vi "Main.vi"(10 "VISA resource name":refnum<visa-resource-name>, 11 "Module Admin":refnum<class "Delacor_lib_QMH_Module Admin.lvclass">) -> ()   [LabVIEW 2018, in "SPIM7_CAM.lvlib"]
doc: "This template is based off of the Queued Message Handler design pattern and the Queued Message Handler project template that ships with LabVIEW.\n\nThe main difference is that the queue is private to this module and communication between modules is performed via Broadcast and Request events.\n\nRequest events are wrapped in public API methods and are handled in the Event Handling Loop (EHL) of this VI. Any module can register for Broadcast events sent by this module. The EHL generates messages based on user interface actions.\n\nThe Message Handling Loop (MHL) processes messages generated by the EHL, or by other messages. The messages are string values, so new messages can be added easily to the Message Cases case structure in the MHL. Each message cluster can also provide an optional value for Message Data, which is a variant that can be converted to whatever message-specific data is required.\n_____\nBased on DQMH Project Template 6.0.0.91."
uses:
  SPIM7_CAM.lvlib
  <vilib>/Delacor/Delacor QMH/Libraries/Module Admin_class/Delacor_lib_QMH_Module Admin.lvclass
  Module Data--cluster.ctl
  <vilib>/Delacor/Delacor QMH/Libraries/Message Queue_class/Delacor_lib_QMH_Message Queue.lvclass/Delacor_lib_QMH_Message Queue.ctl
  Stop Argument--cluster.ctl
  <vilib>/Delacor/Delacor QMH/Libraries/Module Admin_class/Delacor_lib_QMH_Module Admin.lvclass/Delacor_lib_QMH_Module Admin.ctl
  Open COM Argument--cluster.ctl
  Close COM Argument--cluster.ctl
  Read Pan angle Argument--cluster.ctl
  Read Pan angle (Reply Payload)--cluster.ctl
  Read TILT angle Argument--cluster.ctl
  Read TILT angle (Reply Payload)--cluster.ctl
  <vilib>/Utility/miscctls.llb/LVPointTypeDef.ctl
  <vilib>/Delacor/Delacor QMH/Libraries/Message Queue_class/Delacor_lib_QMH_Enqueue Message (Single).vi
  <vilib>/Delacor/Delacor QMH/Libraries/Module Admin_class/Delacor_lib_QMH_Get External Launch.vi
  <vilib>/Utility/error.llb/Error Cluster From Error Code.vi
  <vilib>/Instr/_visa.llb/VISA Configure Serial Port (Instr).vi
  <vilib>/ErrorRing/Error Ring.xnode
  <vilib>/Delacor/Delacor QMH/Libraries/Message Queue_class/Delacor_lib_QMH_Message Queue.lvclass
panel:
  out "error out":errorcluster
  out "Status":string
  in  "Simulate MHL Error":bool
  in  "Simulate EHL Error":bool
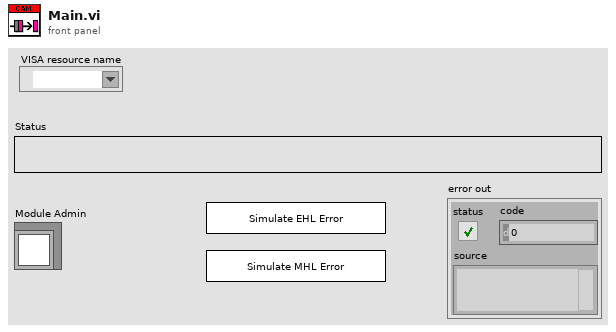
[diagram p1: front panel]
types:
  T1 = typedef "SPIM7_CAM.lvlib/Request Events--cluster.ctl" = cluster{"Stop Module":refnum<user-event>, "Show Panel":refnum<user-event>, "Hide Panel":refnum<user-event>, "Get Module Execution Status":refnum<user-event>, "Show Diagram":refnum<user-event>, "Open COM":refnum<user-event>, "Close COM":refnum<user-event>, "Read Pan angle":refnum<user-event>, "Read TILT angle":refnum<user-event>}
  T2 = typedef "SPIM7_CAM.lvlib/Module Data--cluster.ctl" = cluster{"Status":string, "VISA resource name":refnum<visa-resource-name>}
  T3 = enum32{"invalid lock state", "Not Locked", "Locked (No Password)", "Password-protected"}
  T4 = typedef "SPIM7_CAM.lvlib/Stop Argument--cluster.ctl" = cluster{"Origin":string, "Exit via Stop Module Req?":bool, "Wait for Module to stop?":bool}
  T5 = typedef "SPIM7_CAM.lvlib/Open COM Argument--cluster.ctl" = cluster{"baudrate":u32}
  T6 = typedef "SPIM7_CAM.lvlib/Close COM Argument--cluster.ctl" = cluster{"Boolean":bool}
  T7 = typedef "SPIM7_CAM.lvlib/Read Pan angle Argument--cluster.ctl" = cluster{"Wait Notifier":refnum<notifier>, "wait for reply":bool}
  T8 = typedef "SPIM7_CAM.lvlib/Read TILT angle Argument--cluster.ctl" = cluster{"Wait Notifier":refnum<notifier>, "wait for reply":bool}
  T9 = typedef "LVPointTypeDef.ctl" = cluster{"Horizontal":i16, "Vertical":i16}
  T10 = enum32{"Invalid", "Standard", "Closed", "Hidden", "Minimized", "Maximized"}
  T11 = typedef "SPIM7_CAM.lvlib/Read Pan angle (Reply Payload)--cluster.ctl" = cluster{"Pan angle":dbl, "Read Pan angle_error":errorcluster}
  T12 = typedef "SPIM7_CAM.lvlib/Read TILT angle (Reply Payload)--cluster.ctl" = cluster{"Tilt angle":dbl, "Read TILT angle_error":errorcluster}
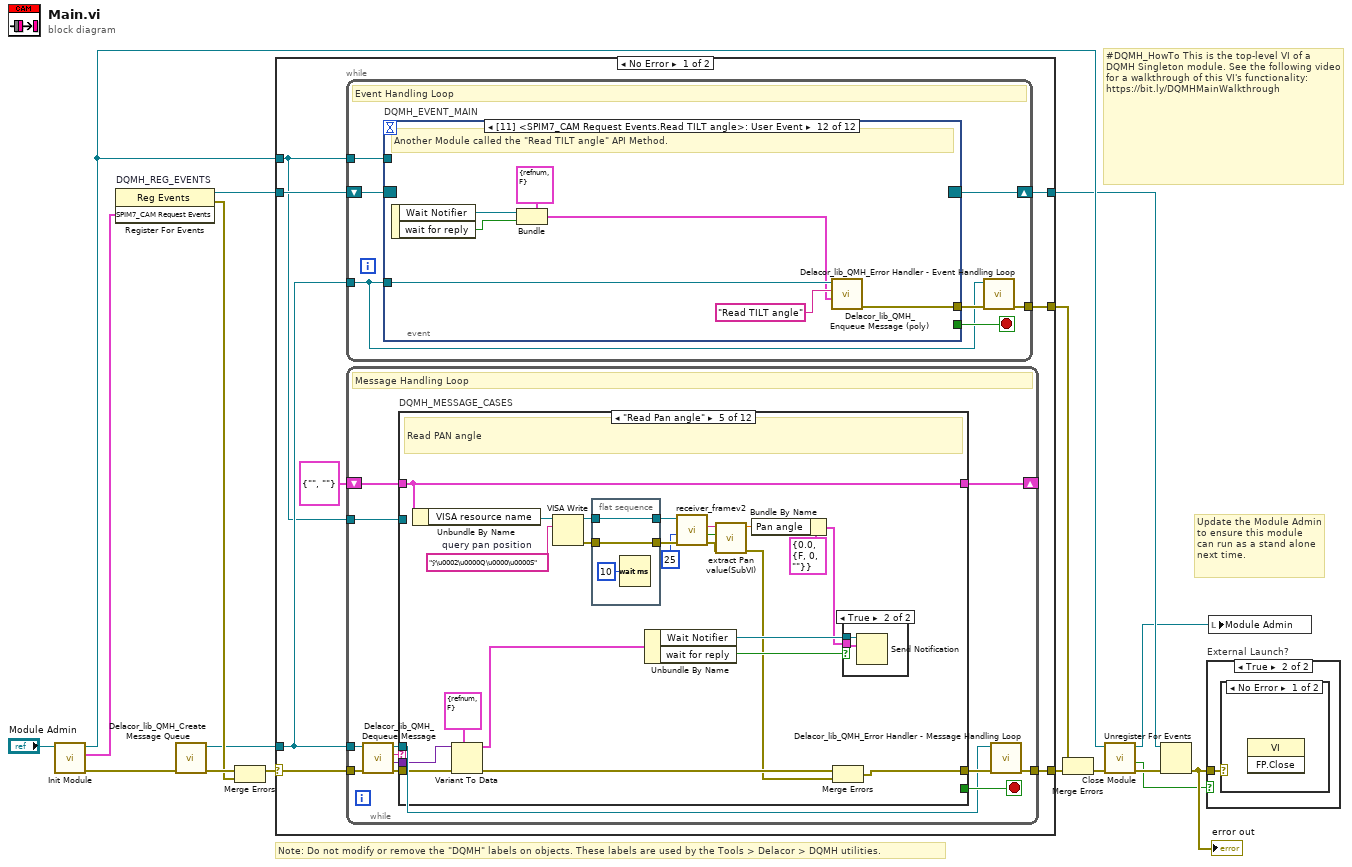
[diagram p0: block diagram]
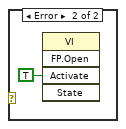
[diagram p3: hidden frame]
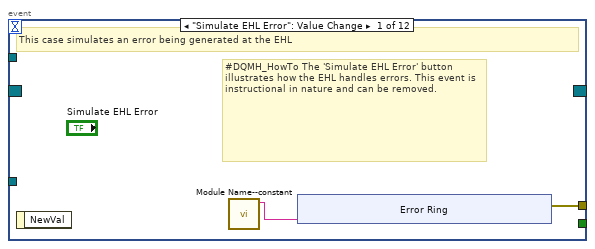
[diagram p4: hidden frame]
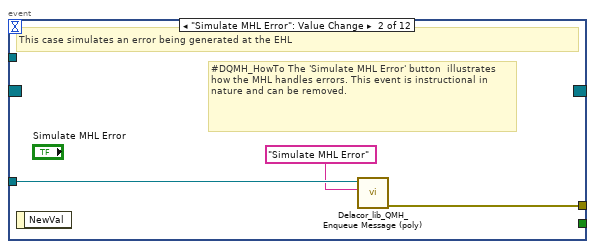
[diagram p5: hidden frame]
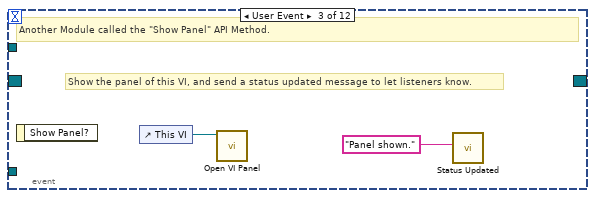
[diagram p6: hidden frame]
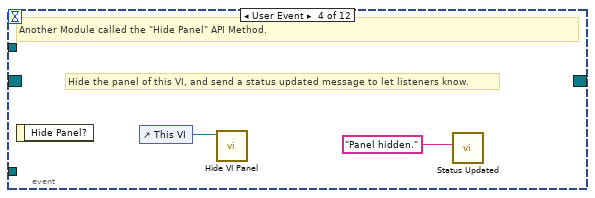
[diagram p7: hidden frame]
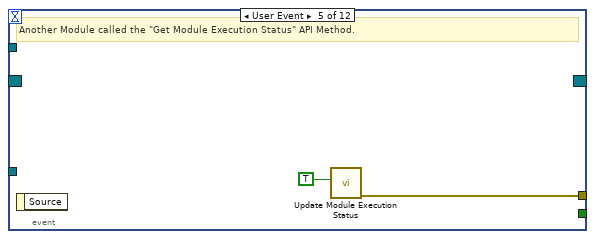
[diagram p8: hidden frame]
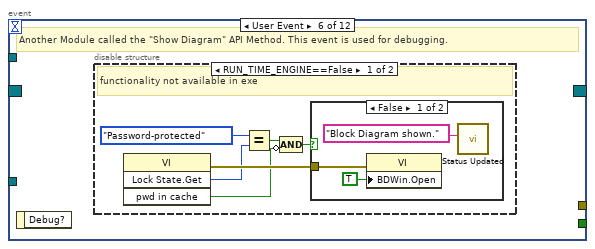
[diagram p9: hidden frame]
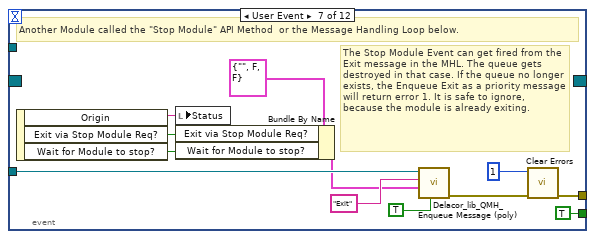
[diagram p12: hidden frame]
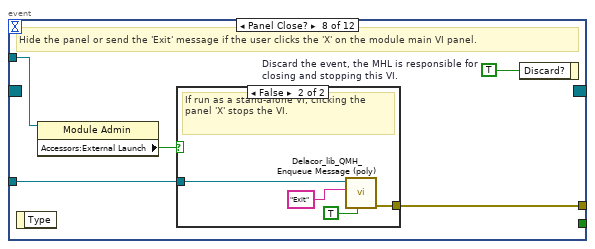
[diagram p13: hidden frame]
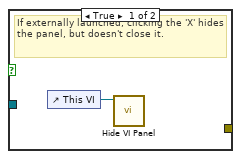
[diagram p14: hidden frame]
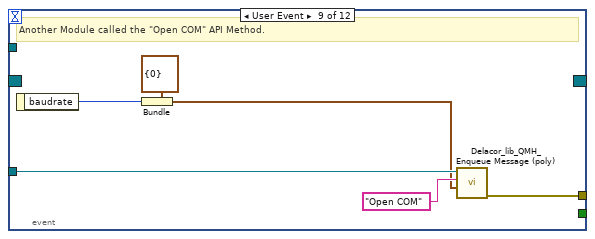
[diagram p15: hidden frame]
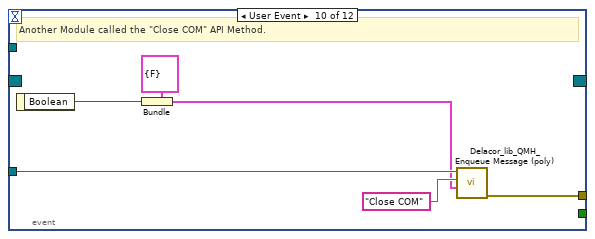
[diagram p16: hidden frame]
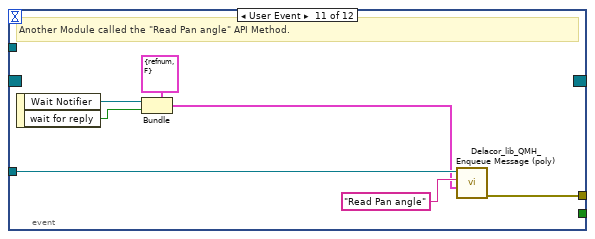
[diagram p17: hidden frame]
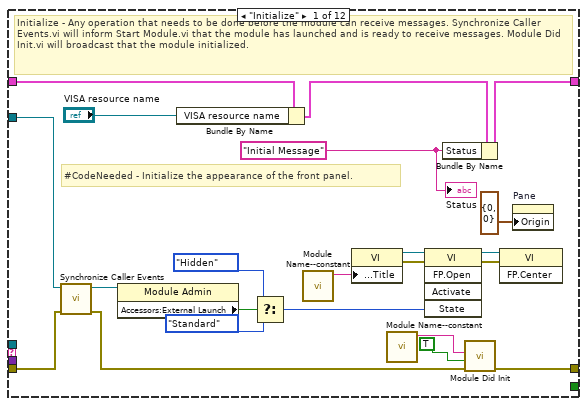
[diagram p18: hidden frame]
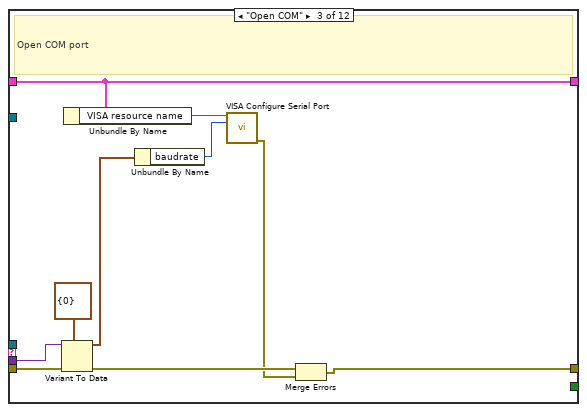
[diagram p20: hidden frame]
diagram:
  # "#DQMH_HowTo This is the top-level VI of a DQMH Singleton module. See the following video for a walkthrough of this VI's functionality: https://bit.ly/DQMHMainWalkthrough"
  # "Note: Do not modify or remove the \"DQMH\" labels on objects. These labels are used by the Tools > Delacor > DQMH utilities."
  # "Update the Module Admin to ensure this module can run as a stand alone next time."
  n1 = call "Init Module.vi"("Singleton Module Admin in"="Module Admin") -> ("error out"=w16:errorcluster, "SPIM7_CAM Request Events"=w5:T1, "Singleton Module Admin out"=w8:refnum<class "Delacor_lib_QMH_Module Admin.lvclass">)  [unwired: 8 in]
  n2 = register-events "DQMH_REG_EVENTS"(w5) -> (reference out=w6:refnum<event-registration>, error out=w9:errorcluster)  [unwired: 2 in]
  n3 = call <vilib>:"Delacor_lib_QMH_Create Message Queue.vi"("error in"=w16) -> ("error out"=w11:errorcluster, "Message Queue"=w4:refnum<class "Delacor_lib_QMH_Message Queue.lvclass">)  [unwired: 9 in]
  n4 = Merge Errors(w11, w9) -> (w10:errorcluster)
  n5 = case shown="No Error" w10 {
    selector: w10 -> [w23 w282]
    tunnel: [w25 w281] -> w17
    tunnel: [w22 w287] -> w7
    tunnel: w6 -> [w20 w287]
    tunnel: w4 -> [w19 w280]
    tunnel: [w24 _] -> w14
    tunnel: w8 -> [w18 w283]
    frame No Error {
      n6 = while {
        tunnel: w19 -> [w26]
        shift-right: [w29] -> w22
        shift-left: w20 -> [w30]
        tunnel: [w31] -> w24
        tunnel: w18 -> [w27]
        stop <- w28 stop-if-true
        # "Event Handling Loop"
        n7 = event "DQMH_EVENT_MAIN" shown="[11] <SPIM7_CAM Request Events.Read TILT angle>: User Event" {
          selector: w30 -> [_ _ _ _ _ _ _ _ _ _ _ _]
          dyn-events: [_ _ _ _ _ _ _ _ _ _ _ _] -> w29
          timeout: _ -> [_ _ _ _ _ _ _ _ _ _ _ _]
          tunnel: [_ _ _ _ _ _ TRUE ("Discard?") _ _ _ _ _] -> w28
          tunnel: w26 -> [_ w43 _ _ _ _ w67 w74 w87 w93 w100 w107]
          tunnel: [w34 w44 _ _ w50 _ w70 w76 w82 w88 w94 w101] -> w32
          tunnel: w27 -> [_ _ _ _ _ _ _ w73 _ _ _ _]
          event "Simulate EHL Error": Value Change {
            # "#DQMH_HowTo The 'Simulate EHL Error' button  illustrates how the EHL handles errors. This event is instructional in nature and can be removed."
            # "This case simulates an error being generated at the EHL"
            n8 = event-data() -> ()  [unwired: 1 in, 1 out]
            n9 = call "Module Name--constant.vi"() -> ("Module Name"=w33:string)  [unwired: 11 in]
            n10 = xnode "Error Ring"("parameter 0"=w33) -> ("error out"=w34:errorcluster)
          }
          event "Simulate MHL Error": Value Change {
            # "#DQMH_HowTo The 'Simulate MHL Error' button  illustrates how the MHL handles errors. This event is instructional in nature and can be removed."
            # "This case simulates an error being generated at the EHL"
            n11 = event-data() -> ()  [unwired: 1 in, 1 out]
            n12 = call-poly <vilib>:"Delacor_lib_QMH_Enqueue Message (poly).vi"("Message"="Simulate MHL Error", "Message Queue in"=w43) -> ("error out"=w44:errorcluster)  [unwired: 8 in, 1 out]
          }
          event User Event {
            # "Show the panel of this VI, and send a status updated message to let listeners know."
            # "Another Module called the \"Show Panel\" API Method."
            n13 = event-data() -> ()  [unwired: 1 in, 1 out]
            n14 = control-ref of="This VI"() -> (w46:refnum<vi>)
            n15 = call "Open VI Panel.vi"("VI"=w46) -> ()  [unwired: 10 in, 1 out]
            n16 = call "Status Updated.vi"("Status"="Panel shown." ("format string")) -> ()  [unwired: 10 in, 1 out]
          }
          event User Event {
            # "Hide the panel of this VI, and send a status updated message to let listeners know."
            # "Another Module called the \"Hide Panel\" API Method."
            n17 = event-data() -> ()  [unwired: 1 in, 1 out]
            n18 = control-ref of="This VI"() -> (w48:refnum<vi>)
            n19 = call "Hide VI Panel.vi"("VI"=w48) -> ()  [unwired: 10 in, 1 out]
            n20 = call "Status Updated.vi"("Status"="Panel hidden." ("format string")) -> ()  [unwired: 10 in, 1 out]
          }
          event User Event {
            # "Another Module called the \"Get Module Execution Status\" API Method."
            n21 = event-data() -> ()  [unwired: 1 in, 1 out]
            n22 = call "Update Module Execution Status.vi"("Running?"=TRUE) -> ("error out"=w50:errorcluster)  [unwired: 10 in]
          }
          event User Event {
            # "Another Module called the \"Show Diagram\" API Method. This event is used for debugging."
            n23 = event-data() -> ()  [unwired: 1 in, 1 out]
            n24 = disable-structure shown="RUN_TIME_ENGINE==False" {
              frame condition #0 (active) {
                # "functionality not available in exe"
                n25 = invoke class="VI" method="Lock State.Get"() -> (error out=w56:errorcluster, "Get Lock State"=w55:T3, "pwd in cache"=w52:bool)  [unwired: 4 in, 1 out]
                n26 = Equal?(x=T3."Password-protected", y=w55) -> (x = y?=w53:bool)
                n27 = Compound Arithmetic op=AND(w53, invert w52) -> (w51:bool)
                n28 = case shown="False" w51 {
                  tunnel: w56 -> [w59 _]
                  frame False {
                    n29 = property class="VI"(error in=w59, "BDWin.Open"=TRUE ("Block Diagram Window:Open")) -> ()  [unwired: 1 in, 2 out]
                    n30 = call "Status Updated.vi"("Status"="Block Diagram shown." ("format string")) -> ()  [unwired: 10 in, 1 out]
                  }
                  frame True {
                    # "Password-protected VI, and the password is not in the cache. Do not show the diagram."
                  }
                }
              }
              frame condition #1 {
              }
            }
          }
          event User Event {
            # "The Stop Module Event can get fired from the Exit message in the MHL. The queue gets destroyed in that case. If the queue no longer exists, the Enqueue Exit as a priority message will return error 1. It is safe to ignore, because the module is already exiting."
            # "Another Module called the \"Stop Module\" API Method  or the Message Handling Loop below."
            n31 = event-data() -> ("Origin"=w66:string, "Exit via Stop Module Req?"=w62:bool, "Wait for Module to stop?"=w61:bool)  [unwired: 1 in]
            n32 = local write "Status"(w66) -> ()
            n33 = Bundle By Name(cluster=T4 {"Origin"="", "Exit via Stop Module Req?"=FALSE, "Wait for Module to stop?"=FALSE} ("Stop Argument"), "Exit via Stop Module Req?"=w62, "Wait for Module to stop?"=w61) -> (w60:T4)
            n34 = call-poly <vilib>:"Delacor_lib_QMH_Enqueue Message (poly).vi"("Priority Message? (F)"=TRUE, "Message Data"=w60, "Message"="Exit", "Message Queue in"=w67) -> ("error out"=w71:errorcluster)  [unwired: 6 in, 1 out]
            n35 = call <vilib>:"Clear Errors.vi"("error in (no error)"=w71, "specific error code to clear (0: all)"=1) -> ("error out"=w70:errorcluster)  [unwired: 4 in, 1 out]
          }
          event Panel Close? {
            w75 = TRUE  # Discard the event, the MHL is responsible for closing and stopping this VI.
            # "Hide the panel or send the 'Exit' message if the user clicks the 'X' on the module main VI panel."
            n36 = event-data() -> ()  [unwired: 1 in, 1 out]
            n37 = property class="Module Admin"(reference=w73) -> ("Accessors:External Launch"=w72:bool)  [unwired: 1 in, 2 out]
            n38 = case shown="False" w72 {
              tunnel: w74 -> [_ w80]
              tunnel: [_ w81] -> w76
              frame True {
                # "If externally launched, clicking the 'X' hides the panel, but doesn't close it."
                n39 = control-ref of="This VI"() -> (w77:refnum<vi>)
                n40 = call "Hide VI Panel.vi"("VI"=w77) -> ()  [unwired: 10 in, 1 out]
              }
              frame False {
                # "If run as a stand-alone VI, clicking the panel 'X' stops the VI."
                n41 = call-poly <vilib>:"Delacor_lib_QMH_Enqueue Message (poly).vi"("Priority Message? (F)"=TRUE, "Message"="Exit", "Message Queue in"=w80) -> ("error out"=w81:errorcluster)  [unwired: 7 in, 1 out]
              }
            }
            n42 = event-data("Discard?"=w75) -> ()  [unwired: 1 in, 1 out]
          }
          event User Event {
            # "Another Module called the \"Open COM\" API Method."
            n43 = event-data() -> ("baudrate"=w83:u32)  [unwired: 1 in]
            n44 = Bundle(cluster=T5 {"baudrate"=0} ("Open COM Argument"), "baudrate"=w83) -> (w84:T5)
            n45 = call-poly <vilib>:"Delacor_lib_QMH_Enqueue Message (poly).vi"("Message Data"=w84, "Message"="Open COM", "Message Queue in"=w87) -> ("error out"=w82:errorcluster)  [unwired: 7 in, 1 out]
          }
          event User Event {
            # "Another Module called the \"Close COM\" API Method."
            n46 = event-data() -> ("Boolean"=w89:bool)  [unwired: 1 in]
            n47 = Bundle(cluster=T6 {"Boolean"=FALSE} ("Close COM Argument"), "Boolean"=w89) -> (w90:T6)
            n48 = call-poly <vilib>:"Delacor_lib_QMH_Enqueue Message (poly).vi"("Message Data"=w90, "Message"="Close COM", "Message Queue in"=w93) -> ("error out"=w88:errorcluster)  [unwired: 7 in, 1 out]
          }
          event User Event {
            # "Another Module called the \"Read Pan angle\" API Method."
            n49 = event-data() -> ("Wait Notifier"=w96:refnum<notifier>, "wait for reply"=w95:bool)  [unwired: 1 in]
            n50 = Bundle(cluster=T7 {"Wait Notifier"=refnum, "wait for reply"=FALSE} ("Read Pan angle Argument"), "Wait Notifier"=w96, "wait for reply"=w95) -> (w97:T7)
            n51 = call-poly <vilib>:"Delacor_lib_QMH_Enqueue Message (poly).vi"("Message Data"=w97, "Message"="Read Pan angle", "Message Queue in"=w100) -> ("error out"=w94:errorcluster)  [unwired: 7 in, 1 out]
          }
          event User Event {
            # "Another Module called the \"Read TILT angle\" API Method."
            n52 = event-data() -> ("Wait Notifier"=w103:refnum<notifier>, "wait for reply"=w102:bool)  [unwired: 1 in]
            n53 = Bundle(cluster=T8 {"Wait Notifier"=refnum, "wait for reply"=FALSE} ("Read TILT angle Argument"), "Wait Notifier"=w103, "wait for reply"=w102) -> (w104:T8)
            n54 = call-poly <vilib>:"Delacor_lib_QMH_Enqueue Message (poly).vi"("Message Data"=w104, "Message"="Read TILT angle", "Message Queue in"=w107) -> ("error out"=w101:errorcluster)  [unwired: 7 in, 1 out]
          }
        }
        n55 = call-dynamic "Delacor_lib_QMH_Error Handler - Event Handling Loop.vi"("error in"=w32, "Message Queue in"=w26) -> ("dup error in"=w31:errorcluster)  [unwired: 8 in, 1 out]
      }
      n56 = while {
        tunnel: w19 -> [w110]
        shift-right: [w114] -> _
        shift-left: T2 {"Status"="", "VISA resource name"=""} ("Data Cluster") -> [w115]
        tunnel: w23 -> [w118]
        tunnel: [w116] -> w25
        tunnel: w18 -> [w108]
        stop <- w113 stop-if-true
        # "Message Handling Loop"
        n57 = call-dynamic "Delacor_lib_QMH_Dequeue Message.vi"("error in"=w118, "Message Queue in"=w110) -> ("error out"=w117:errorcluster, "Message Data"=w111:variant, "Message"=w112:string, "Message Queue out"=w109:refnum<class "Delacor_lib_QMH_Message Queue.lvclass">)  [unwired: 6 in]
        n58 = case "DQMH_MESSAGE_CASES" shown="\"Read Pan angle\"" w112 {
          selector: w112 -> [_ _ _ _ _ _ _ _ _ _ _ w267]
          tunnel: w109 -> [_ _ _ _ _ _ _ _ _ w237 w259 _]
          tunnel: w117 -> [w139 w143 w153 w161 w184 w212 w220 w222 w227 w244 w265 w269]
          tunnel: [w137 w143 w145 w155 w176 w203 w219 w222 w226 w240 w262 w270] -> w119
          tunnel: w115 -> [w120 w142 w148 w157 w173 w202 w218 w221 w224 w239 w258 w268]
          tunnel: [w128 w142 w148 w157 w173 w202 w218 w221 w224 w239 w258 w268] -> w114
          tunnel: [_ _ _ _ _ _ _ _ _ _ w257 _] -> w113
          tunnel: w111 -> [_ _ w151 w159 w182 w210 _ _ _ w238 w256 _]
          tunnel: w108 -> [w129 _ _ _ _ _ _ _ _ w236 w251 _]
          frame "Initialize" {
            w124 = "Initial Message" ("Initial Message")
            # "#CodeNeeded - Initialize the appearance of the front panel."
            # "Initialize - Any operation that needs to be done before the module can receive messages. Synchronize Caller Events.vi will inform Start Module.vi that the module has launched and is ready to receive messages. Module Did Init.vi will broadcast that the module initialized."
            n59 = call "Synchronize Caller Events.vi"("error in (no error)"=w139, "Singleton Module Admin in"=w129) -> ("error out"=w138:errorcluster, "Singleton Module Admin out"=w125:refnum<class "Delacor_lib_QMH_Module Admin.lvclass">)  [unwired: 8 in]
            n60 = property class="Module Admin"(reference=w125) -> ("Accessors:External Launch"=w133:bool)  [unwired: 1 in, 2 out]
            n61 = Bundle By Name(cluster=w120, "VISA resource name"="VISA resource name") -> (w121:T2)
            n62 = Select(t=T10."Hidden" ("State"), s=w133, f=T10."Standard" ("State")) -> (s? t:f=w130:T10)
            n63 = call "Module Name--constant.vi"() -> ("Module Name"=w136:string)  [unwired: 11 in]
            n64 = property class="VI"("Front Panel.Title"=w136) -> (reference out=w135:refnum<vi>, error out=w141:errorcluster)  [unwired: 2 in]
            n65 = call "Module Name--constant.vi"() -> ("Module Name"=w126:string)  [unwired: 11 in]
            n66 = invoke class="VI" method="FP.Open"(reference=w135, error in=w141, "State"=w130) -> (reference out=w134:refnum<vi>, error out=w140:errorcluster)  [unwired: 2 in, 3 out]
            n67 = Bundle By Name(cluster=w121, "Status"=w124) -> (w128:T2)
            n68 = call "Module Did Init.vi"("error in (no error)"=w138, "Initialized?"=TRUE, "Origin"=w126) -> ("error out"=w137:errorcluster)  [unwired: 8 in]
            n69 = invoke class="VI" method="FP.Center"(reference=w134, error in=w140) -> ()  [unwired: 1 in, 3 out]
            n70 = property on="Pane" class="Pane"("Origin"=T9 {"Horizontal"=0, "Vertical"=0}) -> ()  [unwired: 2 in, 2 out]
            "Status" <- w124
          }
          frame "---Module Specific---" {
            # "Separator -- The following cases handle messages specific to this Module."
          }
          frame "Open COM" {
            # "Open COM port"
            n71 = Variant To Data(error in=w153, type=T5 {"baudrate"=0} ("Open COM Argument"), Variant=w151) -> (data=w149:T5, error out=w152:errorcluster)
            n72 = Unbundle By Name(w148) -> ("VISA resource name"=w147:refnum<visa-resource-name>)
            n73 = Unbundle By Name(w149) -> ("baudrate"=w146:u32)
            n74 = call-poly "VISA Configure Serial Port"("VISA resource name"=w147, "baud rate (9600)"=w146) -> ("error out"=w144:errorcluster)  [unwired: 12 in, 1 out]
            n75 = Merge Errors(w152, w144) -> (w145:errorcluster)
          }
          frame "Close COM" {
            # "Close COM port"
            n76 = Unbundle By Name(w157) -> ("VISA resource name"=w156:refnum<visa-resource-name>)
            n77 = Variant To Data(error in=w161, type=T6 {"Boolean"=FALSE} ("Close COM Argument"), Variant=w159) -> (error out=w160:errorcluster)  [unwired: 1 out]
            n78 = VISA Close(VISA resource name=w156) -> (error out=w154:errorcluster)  [unwired: 1 in]
            n79 = Merge Errors(w160, w154) -> (w155:errorcluster)
          }
          frame "Read Pan angle" {
            w167 = "ÿ\u0002\u0000Q\u0000\u0000S"  # query pan position
            # "Read PAN angle"
            n80 = Unbundle By Name(w173) -> ("VISA resource name"=w162:refnum<visa-resource-name>)
            n81 = Variant To Data(error in=w184, type=T7 {"Wait Notifier"=refnum, "wait for reply"=FALSE} ("Read Pan angle Argument"), Variant=w182) -> (data=w180:T7, error out=w183:errorcluster)
            n82 = VISA Write(VISA resource name=w162, write buffer=w167) -> (VISA resource name out=w168:refnum<visa-resource-name>, error out=w170:errorcluster)  [unwired: 1 in, 1 out]
            n83 = flat-sequence {
              tunnel: [w186] -> w171
              tunnel: w170 -> [w186]
              tunnel: [w185] -> w169
              tunnel: w168 -> [w185]
              frame #0 {
                n84 = Wait (ms)(milliseconds to wait=u32 10) -> ()  [unwired: 1 out]
              }
            }
            n85 = Unbundle By Name(w180) -> ("Wait Notifier"=w179:refnum<notifier>, "wait for reply"=w178:bool)
            n86 = call "receiver_framev2.vi"("error in (no error)"=w171, "Timeout(100ms)"=u32 25, "Visa In"=w169) -> ("error out"=w172:errorcluster, "TimeOut?"=w174:bool, "response"=w175:string)  [unwired: 5 in, 1 out]
            n87 = call "extract Pan value(SubVI).vi"("error in (no error)"=w172, "TimeOut"=w174, "response"=w175) -> ("error out"=w163:errorcluster, "pan angle"=w166:dbl)  [unwired: 7 in]
            n88 = Bundle By Name(cluster=T11 {"Pan angle"=0.0, "Read Pan angle_error"={"status"=FALSE, "code"=0, "source"=""}} ("Read Pan angle (Reply Payload)"), "Pan angle"=w166) -> (w165:T11)
            n89 = Merge Errors(w183, w163) -> (w176:errorcluster)
            n90 = case shown="True" w178 {
              tunnel: w179 -> [_ w189]
              tunnel: w165 -> [_ w188]
              frame False {
              }
              frame True {
                n91 = Send Notification(notification=w188, notifier=w189) -> ()  [unwired: 1 in, 2 out]
              }
            }
          }
          frame "Read TILT angle" {
            # "Read TiILT angle"
            n92 = Unbundle By Name(w202) -> ("VISA resource name"=w190:refnum<visa-resource-name>)
            n93 = Variant To Data(error in=w212, type=T8 {"Wait Notifier"=refnum, "wait for reply"=FALSE} ("Read TILT angle Argument"), Variant=w210) -> (data=w208:T8, error out=w211:errorcluster)
            n94 = Unbundle By Name(w208) -> ("Wait Notifier"=w207:refnum<notifier>, "wait for reply"=w206:bool)
            n95 = VISA Write(VISA resource name=w190, write buffer="ÿ\u0002\u0000S\u0000\u0000U") -> (VISA resource name out=w198:refnum<visa-resource-name>, error out=w200:errorcluster)  [unwired: 1 in, 1 out]
            n96 = flat-sequence {
              tunnel: [w214] -> w201
              tunnel: w200 -> [w214]
              tunnel: [w213] -> w199
              tunnel: w198 -> [w213]
              frame #0 {
                n97 = Wait (ms)(milliseconds to wait=u32 10) -> ()  [unwired: 1 out]
              }
            }
            n98 = call "receiver_framev2.vi"("error in (no error)"=w201, "Timeout(100ms)"=u32 25, "Visa In"=w199) -> ("error out"=w192:errorcluster, "TimeOut?"=w194:bool, "response"=w195:string)  [unwired: 5 in, 1 out]
            n99 = call "extract Tilt value(SubVI).vi"("error in (no error)"=w192, "Time out?"=w194, "Pelco-D response"=w195) -> ("error out"=w191:errorcluster, "tilt1"=w193:dbl)  [unwired: 7 in]
            n100 = Merge Errors(w211, w191) -> (w203:errorcluster)
            n101 = Bundle By Name(cluster=T12 {"Tilt angle"=0.0, "Read TILT angle_error"={"status"=FALSE, "code"=0, "source"=""}} ("Read TILT angle (Reply Payload)"), "Tilt angle"=w193) -> (w205:T12)
            n102 = case shown="True" w206 {
              tunnel: w207 -> [_ w217]
              tunnel: w205 -> [_ w216]
              frame False {
              }
              frame True {
                n103 = Send Notification(notification=w216, notifier=w217) -> ()  [unwired: 1 in, 2 out]
              }
            }
          }
          frame "---Copy This Frame---" {
            # "Duplicate this frame when creating new messages.  Change this comment in the duplicated frame to describe this message."
            n104 = Merge Errors(w220) -> (w219:errorcluster)
          }
          frame "---Exit and Error Handling---" {
            # "Separator - The following cases handle errors and exit messages."
          }
          frame "Simulate MHL Error" {
            # "#DQMH_HowTo The 'Simulate MHL Error' button  illustrates how the MHL handles errors. This event is instructional in nature and can be removed."
            # "Simulate an error occurring at the MHL"
            n105 = call "Module Name--constant.vi"() -> ("Module Name"=w223:string)  [unwired: 11 in]
            n106 = xnode "Error Ring"("parameter 0"=w223) -> ("error out"=w225:errorcluster)
            n107 = Merge Errors(w227, w225) -> (w226:errorcluster)
          }
          frame "Error" {
            # "#CodeRecommended - If you ever change the name of this \"Error\" message, you'll need to update the name in the Check Loop Error.vi as well."
            # "#CodeRecommended - If the module is running in standalone mode (External Launch = FALSE), this code will pop up an error dialog and call the 'Exit' message if an error occurs. Add more fine-grained error handling here."
            # "Error - Check the error message data and respond accordingly. This message is sent by the \"Error Handler\" VIs at the end of each loop in this application."
            n108 = property class="Module Admin"(reference=w236) -> ("Accessors:External Launch"=w235:bool)  [unwired: 1 in, 2 out]
            n109 = Variant To Data(error in=w244, type=errorcluster {"status"=FALSE, "code"=0, "source"=""} ("error constant"), Variant=w238) -> (data=w245:errorcluster, error out=w242:errorcluster)
            n110 = call "Error Reported.vi"("Error"=w245) -> ()  [unwired: 10 in, 1 out]
            n111 = case shown="False" w235 {
              tunnel: [w250 _] -> w241
              tunnel: w237 -> [w248 _]
              tunnel: w245 -> [w249 _]
              frame False {
                # "If the module is running standalone, then pop up an error dialog and call the \"Exit\" message."
                n112 = call <vilib>:"Simple Error Handler.vi"("error in (no error)"=w249) -> ()  [unwired: 4 in, 5 out]
                n113 = call-poly <vilib>:"Delacor_lib_QMH_Enqueue Message (poly).vi"("Priority Message? (F)"=TRUE, "Message"="Exit", "Message Queue in"=w248) -> ("error out"=w250:errorcluster)  [unwired: 7 in, 1 out]
              }
              frame True {
                # "If the module was launched externally, calling the Error Reported broadcast VI is the only action performed by the \"Error\" message. The module's caller can then process the error appropriately."
              }
            }
            n114 = Merge Errors(w242, w241) -> (w240:errorcluster)
            n115 = local write "error out"(w240) -> ()
          }
          frame "Exit" {
            w255 = 91  # 91: not all Exit messages will have an argument
            w257 = TRUE  # Stop the VI
            # "Release the message queue reference"
            # "#CodeNeeded - Add any required cleanup code here"
            # "Exit - Exit the application."
            n116 = Variant To Data(error in=w265, type=T4 {"Origin"="", "Exit via Stop Module Req?"=FALSE, "Wait for Module to stop?"=FALSE} ("Stop Argument"), Variant=w256) -> (data=w253:T4, error out=w261:errorcluster)
            n117 = call <vilib>:"Clear Errors.vi"("error in (no error)"=w261, "specific error code to clear (0: all)"=w255) -> ("error out"=w264:errorcluster)  [unwired: 4 in, 1 out]
            n118 = control-ref of="This VI"() -> (w252:refnum<vi>)
            n119 = call-dynamic "Delacor_lib_QMH_Release Message Queue.vi"("error in"=w264, "Message Queue"=w259) -> ("error out"=w263:errorcluster)  [unwired: 9 in]
            n120 = call "Handle Exit.vi"("Stop Argument"=w253, "Admin in"=w251, "VI reference"=w252) -> ("error out"=w260:errorcluster)  [unwired: 7 in, 1 out]
            n121 = Merge Errors(w263, w260) -> (w262:errorcluster)
          }
          frame Default {
            # "'Default' case only runs if there is a message that isn't defined in any of the other cases.  Output a programming error."
            n122 = call "Module Name--constant.vi"() -> ("Module Name"=w266:string)  [unwired: 11 in]
            n123 = xnode "Error Ring"("parameter 0"=w267, "parameter 1"=w266) -> ("error out"=w271:errorcluster)
            n124 = Merge Errors(w269, w271) -> (w270:errorcluster)
          }
        }
        n125 = call-dynamic "Delacor_lib_QMH_Error Handler - Message Handling Loop.vi"("error in"=w119, "Message Queue in"=w109) -> ("dup error in"=w116:errorcluster)  [unwired: 8 in, 1 out]
      }
    }
    frame Error {
      # "Synchronize Caller Events.vi will inform Start Module.vi that the module has launched and will let the code calling Start Module.vi register for broadcasts and would permit the caller receive the broadcast that an error occurred at launch time."
      n126 = call-dynamic "Delacor_lib_QMH_Release Message Queue.vi"("error in"=w282, "Message Queue"=w280) -> ("error out"=w281:errorcluster)  [unwired: 9 in]
      n127 = call "Synchronize Caller Events.vi"("Singleton Module Admin in"=w283) -> ("error out"=w288:errorcluster)  [unwired: 9 in, 1 out]
      n128 = call "Module Name--constant.vi"() -> ("Module Name"=w286:string)  [unwired: 11 in]
      n129 = Format Into String(format string="An error occurred during initialization. %s is no longer running.", w286) -> (resulting string=w284:string)  [unwired: 2 in, 1 out]
      n130 = Merge Errors(w281, w288) -> (w289:errorcluster)
      n131 = call "Error Reported.vi"("Additional Information"=w284, "Error"=w289) -> ()  [unwired: 9 in, 1 out]
    }
  }
  n132 = Merge Errors(w14, w17) -> (w13:errorcluster)
  n133 = call "Close Module.vi"("error in (no error)"=w13, "Module Admin in"=w8) -> ("error out"=w15:errorcluster, "External Launch"=w1:bool, "Module Admin out"=w2:refnum<class "Delacor_lib_QMH_Module Admin.lvclass">)  [unwired: 7 in]
  n134 = Unregister For Events(event registration refnum=w7, error in=w15) -> (error out=w12:errorcluster)
  "error out" <- w12
  n135 = case "External Launch?" shown="True" w1 {
    tunnel: w12 -> [_ w290]
    frame False {
    }
    frame True {
      n136 = case shown="No Error" w290 {
        frame No Error {
          n137 = invoke class="VI" method="FP.Close"() -> ()  [unwired: 3 in, 3 out]
        }
        frame Error {
          n138 = invoke class="VI" method="FP.Open"("Activate"=TRUE ("Activate?")) -> ()  [unwired: 4 in, 5 out]
        }
      }
    }
  }
  n139 = local write "Module Admin"(w2) -> ()
